vi "FindSimilarDataFromArrString.vi"(10 "find str":string, 11 "arr string in":string[](array[string])) -> (3 "result":string[](array[string]))   [LabVIEW 2018, in "Library-DataConvert.lvlib"]
uses:
  Library-DataConvert.lvlib
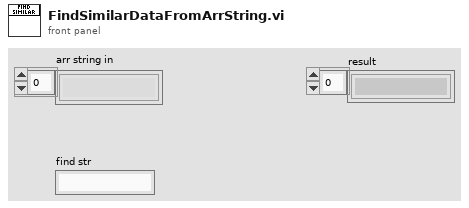
[diagram p1: front panel]
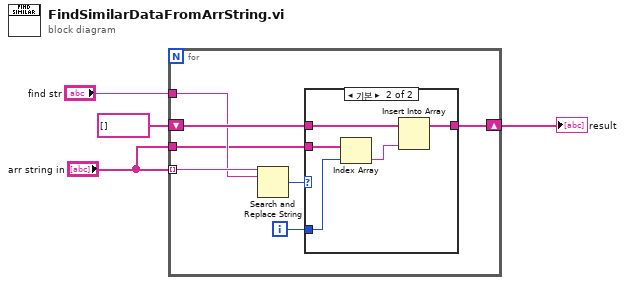
[diagram p0: block diagram]
diagram:
  n1 = for {
    tunnel: "arr string in" -> [w7] mode=indexing
    shift-right: [w8] -> w3
    shift-left: string[] [] ("result") -> [w9]
    tunnel: "find str" -> [w6]
    tunnel: "arr string in" -> [w5]
    i -> [w10]
    n2 = Search and Replace String(input string=w7, search string=w6) -> (number of replacements=w11:i32)  [unwired: 6 in, 3 out]
    n3 = case shown="기본" w11 {
      tunnel: w5 -> [_ w17]
      tunnel: w10 -> [_ w16]
      tunnel: w9 -> [w12 w15]
      tunnel: [w12 w13] -> w8
      frame 0 {
      }
      frame Default {
        n4 = Index Array(array=w17, index=w16) -> (element=w14:string)
        n5 = Insert Into Array(array=w15, new element=w14) -> (w13:string[])  [unwired: 1 in]
      }
    }
  }
  "result" <- w3
